vi "HapticSPM_write.vi"() -> ()   [LabVIEW 2022 SP3]
uses:
  Program Files/National Instruments/LabVIEW 2022/user.lib/Haptic Prog Interface/Haptic Prog Interface.lvlib
  <userlib>/Nanonis Prog Interface V5/Nanonis Prog Interface.lvlib
panel:
  in  "Suggested Settings":bool=TRUE
  out "?":bool=TRUE
  out "Surface":dbl caption="Numeric" format="%#_2p"
  out "Z-Position":dbl caption="Numeric" format="%#_2p"
  out "y":string
  out "x":string
  out "scan data":dbl[][](array[numeric])
  out "2D Picture":picture
  out "Force":dbl(slide) scale=-3.0..3.0
  out "Frame String":string
  in  "Stop":bool
  out "Safe tip":bool
  out "Value":dbl caption="Numeric" format="%#_2p"
  out "Reframed Position (m)":cluster{"x (m)":dbl, "y (m)":dbl, "z (m)":dbl} {"z (m)" format="%.1p"; "y (m)" format="%.1p"; "x (m)" format="%.1p"}
  out "Frame Properties (m)":T1
  in  "Function":string(combo)="0" caption="Combo Box"
  in  "Gain (mm/pm)":dbl=1.0 caption="Numeric" format="%.1g"
  in  "k":dbl=1.0 caption="Numeric" step=0.1 format="%.1g"
  in  "Setpoint":dbl=1e-10 caption="Numeric" step=1e-11 format="%.0p"
  in  "Gain":dbl=1.0 caption="Numeric" format="%.1g"
  out "Click Number":dbl caption="Numeric" format="%#_1g"
  in  "Write Z":bool
  in  "Planing Toggle":bool
  in  "Planing Reset":bool
  in  "Save":bool
  # "Super Ultra Mega Haptic SPM Controller 3000"
  # "Scan Window"
  # "Height"
  # "Signal"
  # "Force"
  # "Force"
  # "Planing"
  # "Surface Scale"
  # "Move pens in all three dimensions to calibrate\nClick \"enter\" to turn off recommended settings"
  # "Z Write"
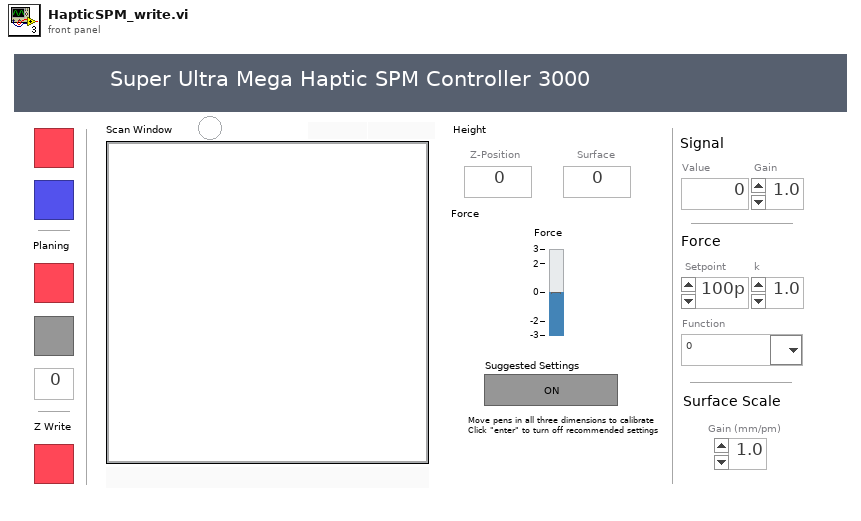
[diagram p1: front panel]
types:
  T1 = cluster{"Center coordinates (m)":cluster{"Xc":sgl, "Yc":sgl}, "Size (m)":cluster{"Width":sgl, "Height":sgl}}
  T2 = cluster{"Fx (N)":dbl, "Fy (N)":dbl, "Fz (N)":dbl}
  T3 = cluster{"kx (N/m)":dbl, "ky (N/m)":dbl, "kz (N/m)":dbl}
  T4 = cluster{"X Drag":bool, "Y Drag":bool, "Z Drag":bool}
  T5 = cluster{"Origin (m)":cluster{"X Origin (m)":dbl, "Y Origin (m)":dbl}, "Frame Size (m)":cluster{"FW (m)":dbl, "FH (m)":dbl}}
  T6 = cluster{"x (mm)":dbl, "y (mm)":dbl, "z (mm)":dbl}
  T7 = typedef "LVBoundsTypeDef.ctl" = cluster{"Width":u32, "Height":u32}
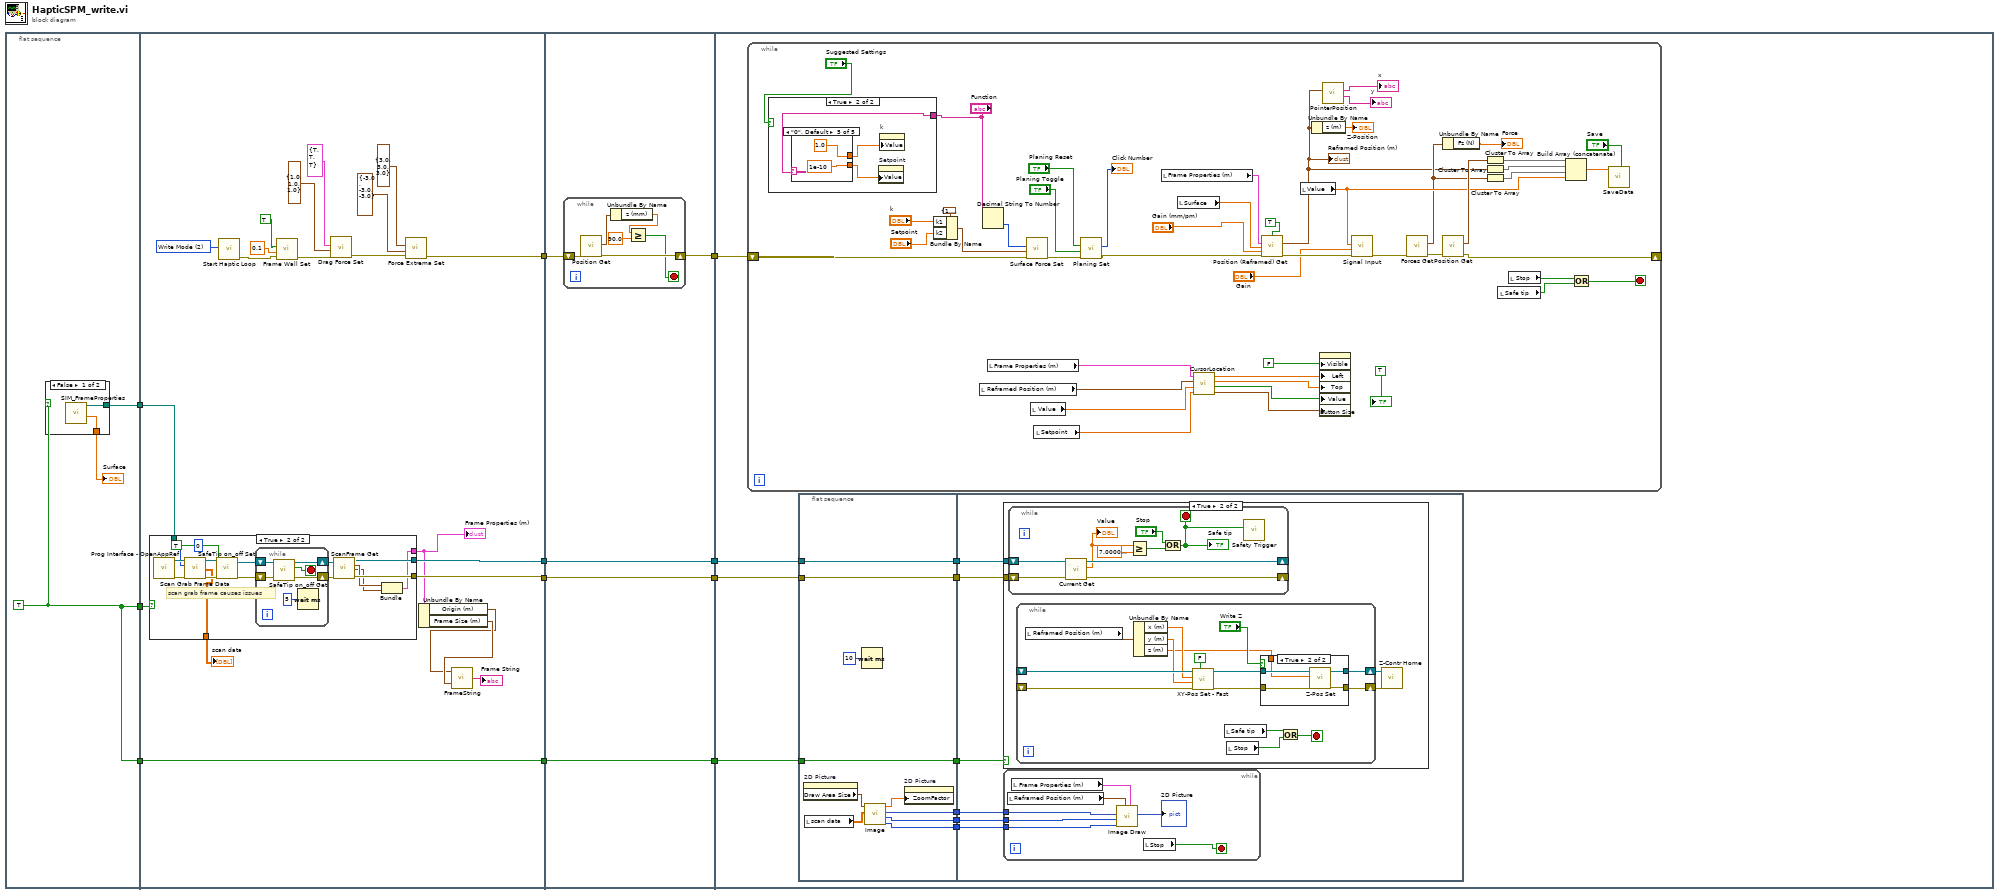
[diagram p0: block diagram]
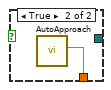
[diagram p2: hidden frame]
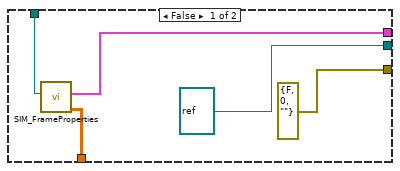
[diagram p3: hidden frame]
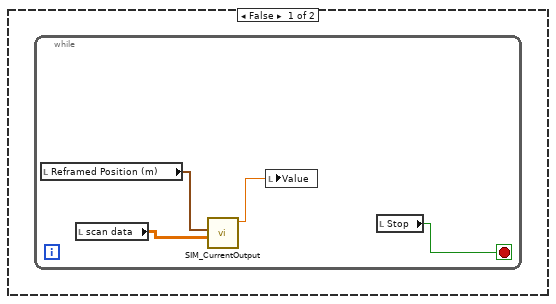
[diagram p4: hidden frame]
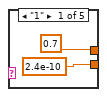
[diagram p7: hidden frame]
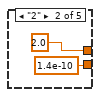
[diagram p8: hidden frame]
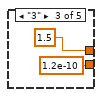
[diagram p9: hidden frame]
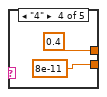
[diagram p10: hidden frame]
diagram:
  n1 = flat-sequence {
    tunnel: [w14] -> w5
    tunnel: [w14] -> w4
    tunnel: [w12] -> w1
    tunnel: [w36] -> w11
    tunnel: [w27] -> w8
    tunnel: [w26] -> w6
    tunnel: w5 -> [w25]
    tunnel: w4 -> [w24]
    tunnel: [w24] -> w3
    tunnel: w1 -> [w18]
    tunnel: w11 -> [w70]
    tunnel: [w69] -> w10
    tunnel: [w68] -> w9
    tunnel: w8 -> [w68]
    tunnel: [w67] -> w7
    tunnel: w6 -> [w67]
    tunnel: w3 -> [w66]
    tunnel: [w66] -> w2
    tunnel: w10 -> [w86]
    tunnel: w9 -> [w84]
    tunnel: w7 -> [w82]
    tunnel: w2 -> [w81]
    frame #0 {
      w14 = TRUE
      n2 = case shown="False" w14 {
        tunnel: [w16 w17] -> w13
        tunnel: [w15 _] -> w12
        frame False {
          n3 = call "SIM_FrameProperties.vi"() -> ("Surf Loc (m)"=w16:dbl, "new file path (Not A Path if cancelled)"=w15:path)  [unwired: 8 in, 2 out]
        }
        frame True {
          n4 = call "AutoApproach.vi"() -> ("Surface Location (m)"=w17:dbl)  [unwired: 11 in]
        }
      }
      "Surface" <- w13
    }
    frame #1 {
      w38 = u16 2 items=["Custom Mode", "Read Mode", "Write Mode"] ("Mode Selection")
      n5 = case shown="True" w25 {
        tunnel: [refnum<vi> refnum ("Application ref out") w54] -> w27
        tunnel: [errorcluster {"status"=FALSE, "code"=0, "source"=""} ("error out") w53] -> w26
        tunnel: [w40 w44] -> w21
        tunnel: [w41 w48] -> w23
        tunnel: w18 -> [w39 _]
        frame False {
          n6 = call "SIM_FrameProperties.vi"("file path (dialog if empty)"=w39) -> ("data"=w41:dbl[][], "Frame Properties (m)"=w40:T5)  [unwired: 7 in, 2 out]
        }
        frame True {
          # "scan grab frame causes issues"
          n7 = call <userlib>:"Prog Interface - OpenAppRef.vi"() -> ("Error out"=w49:errorcluster, "Application reference"=w52:refnum<vi>)  [unwired: 6 in]
          n8 = call <userlib>:"Scan Grab Frame Data.vi"("Application ref in"=w52, "Channel index (0-127)"=u8 0 ("Channel index (0-23)"), "error in (no error)"=w49) -> ("Application ref out"=w51:refnum<vi>, "Scan frame data"=w48:sgl[][], "error out"=w50:errorcluster)  [unwired: 8 in, 2 out]
          n9 = call <userlib>:"SafeTip on_off Set.vi"("error in (no error)"=w50, "SafeTip ON/OFF"=TRUE, "Application ref in"=w51) -> ("error out"=w59:errorcluster, "Application ref out"=w58:refnum<vi>)  [unwired: 7 in]
          n10 = while {
            shift-right: [w63] -> w56
            shift-left: w58 -> [w65]
            shift-right: [w62] -> w55
            shift-left: w59 -> [w64]
            stop <- w60 stop-if-true
            n11 = call <userlib>:"SafeTip on_off Get.vi"("error in (no error)"=w64, "Application ref in"=w65) -> ("error out"=w62:errorcluster, "SafeTip on/off status"=w60:bool, "Application ref out"=w63:refnum<vi>)  [unwired: 7 in]
            n12 = Wait (ms)(milliseconds to wait=u32 5) -> ()  [unwired: 1 out]
          }
          n13 = call <userlib>:"ScanFrame Get.vi"("Application ref in"=w56, "error in (no error)"=w55) -> ("Application ref out"=w54:refnum<vi>, "Center coordinates (m)"=w46:cluster{"Xc":sgl, "Yc":sgl}, "Size (m)"=w45:cluster{"Width":sgl, "Height":sgl}, "error out"=w53:errorcluster)  [unwired: 9 in, 1 out]
          n14 = Bundle("Center coordinates (m)"=w46, "Size (m)"=w45) -> (w44:T1)  [unwired: 1 in]
        }
      }
      "Frame Properties (m)" <- w21
      "scan data" <- w23
      n15 = call "Start Haptic Loop.vi"("Mode Selection"=w38) -> ("error out"=w29:errorcluster)  [unwired: 10 in]
      n16 = call "Frame Wall Set.vi"("error in (no error)"=w29, "Wall Stiffness (N/m)"=0.1 ("Wall Stiffness"), "Restrict to Frame"=TRUE) -> ("error out"=w28:errorcluster)  [unwired: 8 in]
      n17 = call "Drag Force Set.vi"("error in (no error)"=w28, "Drag Coefficients (N/m)"=T3 {"kx (N/m)"=1.0, "ky (N/m)"=1.0, "kz (N/m)"=1.0} ("Drag Coefficients"), "Drag Force Toggles"=T4 {"X Drag"=TRUE, "Y Drag"=TRUE, "Z Drag"=TRUE}) -> ("error out"=w37:errorcluster)  [unwired: 8 in]
      n18 = call "Force Extrema Set.vi"("error in (no error)"=w37, "Minimum Force (N)"=T2 {"Fx (N)"=-3.0, "Fy (N)"=-3.0, "Fz (N)"=-3.0} ("Minimum Force"), "Maximum Force (N)"=T2 {"Fx (N)"=3.0, "Fy (N)"=3.0, "Fz (N)"=3.0} ("Maximum Force")) -> ("error out"=w36:errorcluster)  [unwired: 8 in]
      n19 = Unbundle By Name(w21) -> ("Origin (m)"=w19:cluster{"X Origin (m)":dbl, "Y Origin (m)":dbl}, "Frame Size (m)"=w20:cluster{"FW (m)":dbl, "FH (m)":dbl})
      n20 = call "FrameString.vi"("Size (m)"=w20, "Center coordinates (m)"=w19) -> ("string"=→"Frame String":string)
    }
    frame #2 {
      n21 = while {
        shift-right: [w75] -> w69
        shift-left: w70 -> [w76]
        stop <- w71 stop-if-true
        n22 = call "Position Get.vi"("error in (no error)"=w76) -> ("error out"=w75:errorcluster, "Position"=w74:T6)  [unwired: 9 in]
        n23 = Unbundle By Name(w74) -> ("z (mm)"=w73:dbl)
        n24 = Greater Or Equal?(x=w73, y=90.0) -> (x >= y?=w71:bool)
      }
    }
    frame #3 {
      n25 = while {
        shift-right: [w190] -> _
        shift-left: w86 -> [w196]
        stop <- w150 stop-if-true
        n26 = case shown="True" "Suggested Settings" {
          tunnel: "Function" -> [_ w199]
          frame False {
          }
          frame True {
            n27 = case shown="\"0\", Default" w199 {
              tunnel: [0.7 2.0 1.5 0.4 1.0] -> w198
              tunnel: [2.4e-10 1.4e-10 1.2e-10 8e-11 1e-10] -> w197
              frame "1" {
              }
              frame "2" {
              }
              frame "3" {
              }
              frame "4" {
              }
              frame "0", Default {
              }
            }
            n28 = property on="Setpoint" class="DigNum (strict)"("Value"=w197) -> ()  [unwired: 2 in, 2 out]
            n29 = property on="k" class="DigNum (strict)"("Value"=w198) -> ()  [unwired: 2 in, 2 out]
          }
        }
        n30 = Bundle By Name(cluster=cluster{"k1":dbl, "k2":dbl, "k3":dbl, "k4":dbl} {"k1"=1.0, "k2"=1.0, "k3"=1.0, "k4"=1.0} ("Force Constants"), "k1"="k", "k2"="Setpoint") -> (w183:cluster{"k1":dbl, "k2":dbl, "k3":dbl, "k4":dbl})
        n31 = local read "Reframed Position (m)"() -> (w153:cluster{"x (m)":dbl, "y (m)":dbl, "z (m)":dbl})
        n32 = Decimal String To Number(string="Function") -> (number=w180:i32)  [unwired: 2 in, 1 out]
        n33 = local read "Frame Properties (m)"() -> (w157:T1)
        n34 = call "Surface Force Set.vi"("error in (no error)"=w196, "Force Constants"=w183, "Force Settings"=w180) -> ("error out"=w195:errorcluster)  [unwired: 8 in]
        n35 = local read "Value"() -> (w156:dbl)
        n36 = local read "Setpoint"() -> (w155:dbl)
        n37 = call "Planing Set.vi"("error in (no error)"=w195, "Planing"="Planing Toggle", "Reset"="Planing Reset") -> ("error out"=w186:errorcluster, "Number of Clicks"=→"Click Number":i8)  [unwired: 7 in]
        n38 = local read "Frame Properties (m)"() -> (w168:T1)
        n39 = local read "Surface"() -> (w194:dbl)
        n40 = call "CursorLocation.vi"("Setpoint"=w155, "Value"=w156, "Position (Reframed)"=w153, "Frame Properties (m)"=w157) -> ("Cursor Size"=w158:cluster{"Width":i32, "Height":i32}, "Current Above Setpoint?"=w159:bool, "Y-Coordinate"=w160:dbl, "X-Coordinate"=w161:dbl)
        n41 = call "Position (Reframed) Get.vi"("Z Rescaling"=TRUE, "Frame Properties (m)"=w168, "Surface Location (m)"=w194, "Scaling (mm per pm)"="Gain (mm/pm)", "error in (no error)"=w186) -> ("Reframed Position (m)"=w164:cluster{"x (m)":dbl, "y (m)":dbl, "z (m)":dbl}, "error out"=w192:errorcluster)  [unwired: 9 in]
        "Reframed Position (m)" <- w164
        n42 = local read "Value"() -> (w174:dbl)
        n43 = Unbundle By Name(w164) -> ("z (m)"=→"Z-Position":dbl)
        n44 = property class="Bool (strict)"("Visible"=FALSE, "Left"=w161, "Top"=w160, "Value"=w159, "Button Size"=w158) -> ()  [unwired: 2 in, 2 out]
        n45 = call "PointerPosition.vi"("Reframed Position (m)"=w164) -> ("y string"=→"y":string, "x string"=→"x":string)  [unwired: 9 in]
        n46 = call "Signal Input.vi"("error in (no error)"=w192, "Gain"="Gain", "Signal"=w174) -> ("error out"=w193:errorcluster)  [unwired: 8 in]
        n47 = call "Forces Get.vi"("error in (no error)"=w193) -> ("error out"=w191:errorcluster, "Force (N)"=w169:T2)  [unwired: 9 in]
        n48 = call "Position Get.vi"("error in (no error)"=w191) -> ("error out"=w190:errorcluster, "Position"=w178:T6)  [unwired: 9 in]
        n49 = Unbundle By Name(w169) -> ("Fz (N)"=→"Force":dbl)
        n50 = Cluster To Array(cluster=w178) -> (array=w177:dbl[])
        n51 = Cluster To Array(cluster=w164) -> (array=w176:dbl[])
        n52 = Cluster To Array(cluster=w169) -> (array=w175:dbl[])
        n53 = local read "Safe tip"() -> (w170:bool)
        n54 = local read "Stop"() -> (w171:bool)
        n55 = Build Array (concatenate)(w177, w176, w175, w174) -> (w173:dbl[])
        n56 = Or(x=w171, y=w170) -> (x .or. y?=w150:bool)
        n57 = call "SaveData.vi"("Save"="Save", "Data"=w173) -> ()  [unwired: 10 in]
        "?" <- TRUE
      }
      n58 = flat-sequence {
        tunnel: [w95] -> w85
        tunnel: w84 -> [w95]
        tunnel: [w94] -> w83
        tunnel: w82 -> [w94]
        tunnel: w81 -> [w93]
        tunnel: [w93] -> w80
        tunnel: [w89] -> w79
        tunnel: [w88] -> w78
        tunnel: [w87] -> w77
        tunnel: w85 -> [w102]
        tunnel: w83 -> [w101]
        tunnel: w80 -> [w100]
        tunnel: w79 -> [w99]
        tunnel: w78 -> [w98]
        tunnel: w77 -> [w97]
        frame #0 {
          n59 = property on="2D Picture" class="Pict"() -> ("Draw Area Size"=w92:T7)  [unwired: 2 in, 2 out]
          n60 = local read "scan data"() -> (w90:dbl[][])
          n61 = Wait (ms)(milliseconds to wait=u32 10) -> ()  [unwired: 1 out]
          n62 = call "Image.vi"("data"=w90, "Draw Area Size"=w92) -> ("Rectangle.bottom"=w87:i16, "Rectangle.right"=w88:i16, "new picture"=w89:picture, "ZoomFactor"=w91:dbl)  [unwired: 6 in]
          n63 = property on="2D Picture" class="Pict"("ZoomFactor"=w91) -> ()  [unwired: 2 in, 2 out]
        }
        frame #1 {
          n64 = case shown="True" w100 {
            tunnel: w102 -> [_ w117]
            tunnel: w101 -> [_ w116]
            frame False {
              n65 = while {
                stop <- w111 stop-if-true
                n66 = local read "Reframed Position (m)"() -> (w112:cluster{"x (m)":dbl, "y (m)":dbl, "z (m)":dbl})
                n67 = local read "scan data"() -> (w110:dbl[][])
                n68 = call "SIM_CurrentOutput.vi"("array"=w110, "Position (Reframed)"=w112) -> ("Current Out (A)"=w113:dbl)  [unwired: 8 in, 1 out]
                n69 = local write "Value"(w113) -> ()
                n70 = local read "Stop"() -> (w111:bool)
              }
            }
            frame True {
              n71 = while {
                shift-right: [w124] -> _
                shift-left: w117 -> [w126]
                shift-right: [w123] -> _
                shift-left: w116 -> [w125]
                stop <- w118 stop-if-true
                n72 = call <userlib>:"Current Get.vi"("Error in (no error)"=w125, "Application ref in"=w126) -> ("Error out"=w123:errorcluster, "Current (A)"=w122:sgl, "Application ref out"=w124:refnum<vi>)  [unwired: 5 in]
                "Value" <- w122
                n73 = Greater Or Equal?(x=w122, y=sgl 7e-10) -> (x >= y?=w120:bool)
                n74 = Or(x="Stop", y=w120) -> (x .or. y?=w118:bool)
                "Safe tip" <- w118
                n75 = call "Safety Trigger.vi"("Safety Trigger"=w118) -> ()  [unwired: 9 in, 2 out]
              }
              n76 = while {
                shift-right: [w134] -> w115
                shift-left: _ -> [w140]
                shift-right: [w132] -> w114
                shift-left: _ -> [w141]
                stop <- w127 stop-if-true
                n77 = local read "Reframed Position (m)"() -> (w139:cluster{"x (m)":dbl, "y (m)":dbl, "z (m)":dbl})
                n78 = Unbundle By Name(w139) -> ("x (m)"=w138:dbl, "y (m)"=w137:dbl, "z (m)"=w130:dbl)
                n79 = call <userlib>:"XY-Pos Set - Fast.vi"("Wait end-of-motion (T=True)"=FALSE, "error in (no error)"=w141, "Y (m)"=w137, "X (m)"=w138, "Application ref in"=w140) -> ("error out"=w131:errorcluster, "Application ref out"=w133:refnum<vi>)  [unwired: 4 in]
                n80 = local read "Safe tip"() -> (w129:bool)
                n81 = local read "Stop"() -> (w128:bool)
                n82 = case shown="True" "Write Z" {
                  tunnel: [w143 w146] -> w134
                  tunnel: w133 -> [w143 w148]
                  tunnel: [w142 w145] -> w132
                  tunnel: w131 -> [w142 w147]
                  tunnel: w130 -> [_ w144]
                  frame False {
                  }
                  frame True {
                    n83 = call <userlib>:"Z-Pos Set.vi"("error in (no error)"=w147, "Z position (m)"=w144, "Application ref in"=w148) -> ("error out"=w145:errorcluster, "Application ref out"=w146:refnum<vi>)  [unwired: 7 in]
                  }
                }
                n84 = Or(x=w129, y=w128) -> (x .or. y?=w127:bool)
              }
              n85 = call <userlib>:"Z-Contr Home.vi"("Error in (no error)"=w114, "Application ref in"=w115) -> ()  [unwired: 8 in, 2 out]
            }
          }
          n86 = while {
            tunnel: w99 -> [w108]
            tunnel: w98 -> [w107]
            tunnel: w97 -> [w106]
            stop <- w109 stop-if-true
            n87 = local read "Reframed Position (m)"() -> (w105:cluster{"x (m)":dbl, "y (m)":dbl, "z (m)":dbl})
            n88 = local read "Frame Properties (m)"() -> (w104:T1)
            n89 = call "Image Draw.vi"("Frame Properties (m)"=w104, "Reframed Position (m)"=w105, "ih"=w106, "iw"=w107, "picture"=w108) -> ("new picture"=→"2D Picture":picture)  [unwired: 6 in]
            n90 = local read "Stop"() -> (w109:bool)
          }
        }
      }
    }
  }
